vi "Shared Binary Version.vi"(8 "error in (no error)":errorcluster) -> (0 "error out":errorcluster, 3 "Version":string)   [LabVIEW 2020, in "feature_detection.lvlib" / "Text Tesseract.lvclass"]
doc: "Get the version of the shared binary file for this component."
uses:
  Text Tesseract.lvclass
  common/common.lvlib
  common/bin/gartoolkit_tesseract_32-1.dll
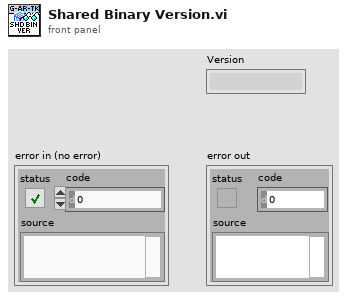
[diagram p1: front panel]
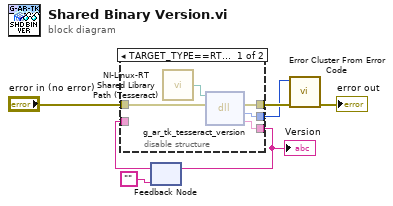
[diagram p0: block diagram]
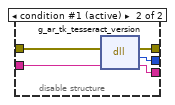
[diagram p2: hidden frame]
diagram:
  n1 = feedback #1("") -> (w5:string)
  n2 = disable-structure "Conditional Disable Structure" shown="TARGET_TYPE==RT&&OS==Linux" {
    disable-tunnel: [w10 w17] -> w3
    disable-tunnel: [w9 w16] -> w2
    disable-tunnel: [w8 w15] -> w6
    disable-tunnel: "error in (no error)" -> [w11 w14]
    disable-tunnel: w5 -> [_ w13]
    frame condition #0 {
      n3 = call "NI-Linux-RT Shared Library Path (Tesseract).vi"() -> ("Path"=w12:path)
      n4 = dll-call lib="?" fn="g_ar_tk_tesseract_version" ("g_ar_toolkit.*.*:g_ar_tk_capture_context_create")(path in=w12, error in=w11) -> (error out=w10:errorcluster, "return type"=w9:i32, "Version"=w8:string)  [unwired: 2 in, 1 out]
    }
    frame condition #1 (active) {
      n5 = dll-call lib="C:/serenial/lib/g-augmented-reality-toolkit/LabVIEW/common/bin/gartoolkit_tesseract_*-1.*" fn="g_ar_tk_tesseract_version" ("g_ar_toolkit.*.*:g_ar_tk_capture_context_create")(error in=w14, "Version"=w13) -> (error out=w17:errorcluster, "return type"=w16:i32, "Version"=w15:string)  [unwired: 2 in, 1 out]
    }
  }
  "Version" <- w6
  n6 = feedback-in #1(w6) -> ()
  n7 = call <vilib>:"Error Cluster From Error Code.vi"("error in (no error)"=w3, "error code (0)"=w2) -> ("error out"=→"error out":errorcluster)  [unwired: 7 in]
